vi "draw the stage.vi"(9 "angle":refnum<vi>, 10 "current pos...":refnum<vi>, 11 "XY Graph 2":refnum<vi>) -> ()   [LabVIEW 2018]
uses:
  cursor action.ctl
  generate linear region.vi
panel:
  out "angle 2":dbl(slide)=743.9484386624194 scale=-90.0..90.0 scale format="%^#6_6g"
  out "current pos...  2":dbl(slide) scale=0.0..16000.0
  in  "XY Graph":cluster{dbl[], dbl[]}[](graph)
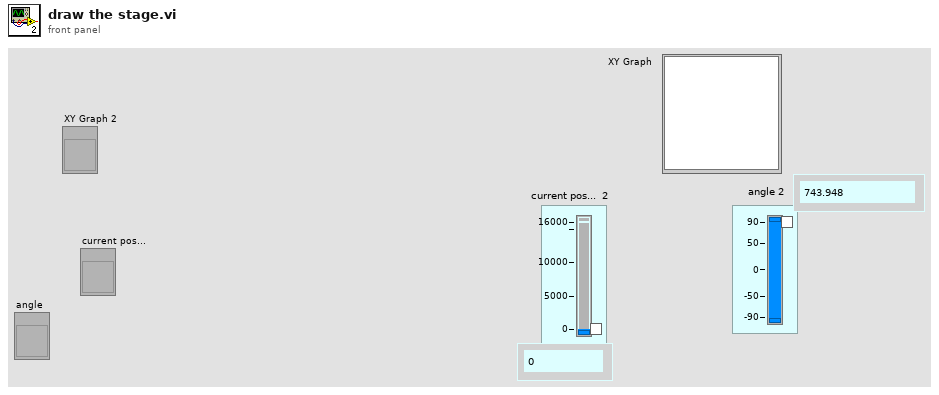
[diagram p1: front panel]
types:
  T1 = typedef "cursor action.ctl" = enum16{"range", "read", "write", "check", "zoom out", "smart zoom out", "zoom to aspect ratio 1", "zoom to win", "zoom out 20%", "zoom in 20%", "-empty", "smart zoom out&aspect", "move range left 20%", "move range right 20%", "move range up 20%", "move range down 20%", "zoom to X win", "zoom to Y win", "zoom out X", "zoom out Y", "zoom in X", "zoom in Y", "check plot scale"}
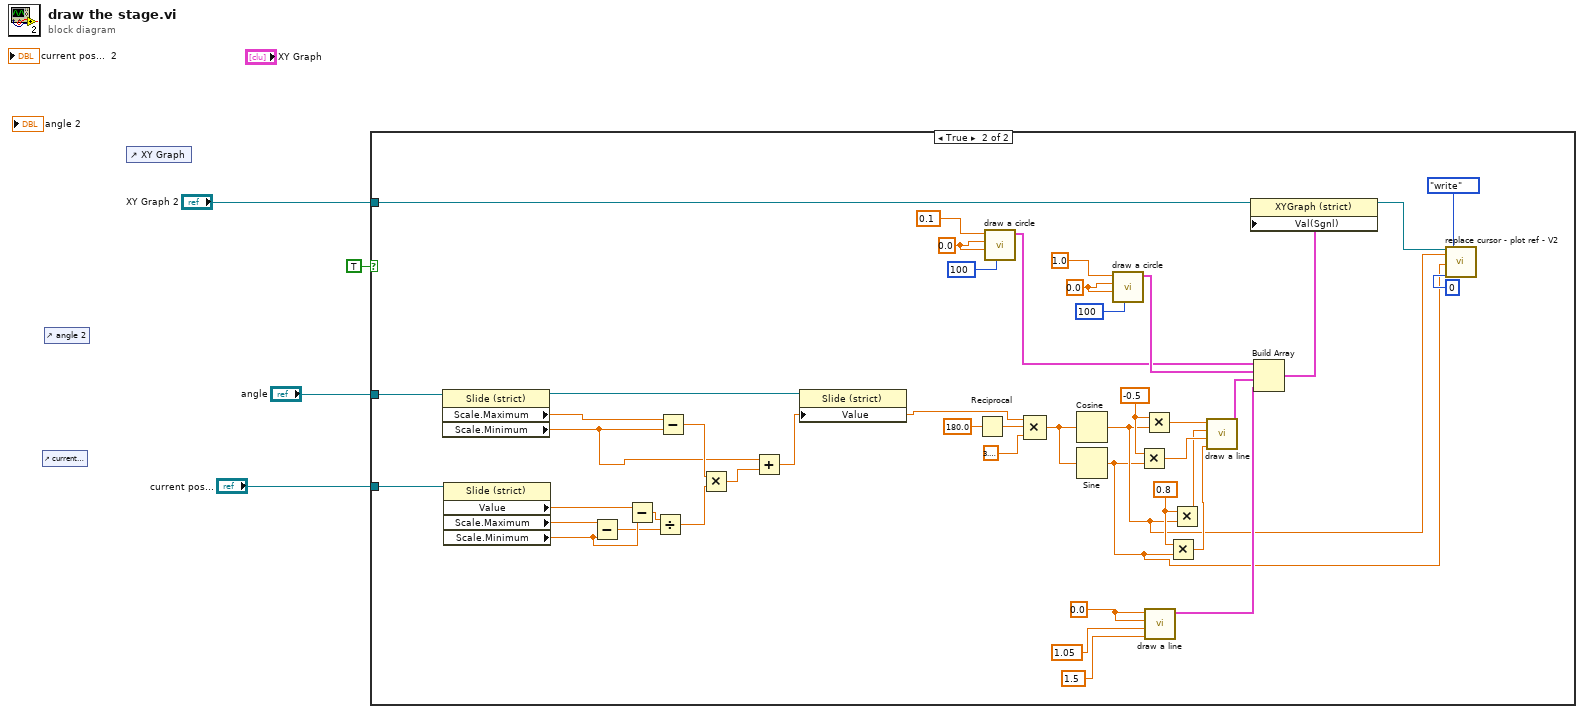
[diagram p0: block diagram]
diagram:
  n1 = control-ref of="current pos...  2"() -> ()  [unwired: 1 out]
  n2 = control-ref of="angle 2"() -> ()  [unwired: 1 out]
  n3 = control-ref of="XY Graph"() -> ()  [unwired: 1 out]
  n4 = case shown="True" TRUE {
    tunnel: "angle" -> [_ w47]
    tunnel: "current pos..." -> [_ w46]
    tunnel: "XY Graph 2" -> [_ w9]
    frame False {
    }
    frame True {
      w13 = 0.0 ("center x")
      w21 = 0.8 ("x")
      w23 = -0.5 ("x")
      w32 = 0.0 ("x0")
      w35 = 0.0 ("center x")
      n5 = property class="Slide (strict)"(reference=w47) -> (reference out=w36:refnum<vi>, "Scale.Maximum"=w40:dbl, "Scale.Minimum"=w14:dbl)  [unwired: 1 in, 1 out]
      n6 = property class="Slide (strict)"(reference=w46) -> ("Value"=w44:dbl, "Scale.Maximum"=w45:dbl, "Scale.Minimum"=w43:dbl)  [unwired: 1 in, 2 out]
      n7 = Subtract(x=w45, y=w43) -> (x-y=w41:dbl)
      n8 = Subtract(x=w44, y=w43) -> (x-y=w42:dbl)
      n9 = Divide(x=w42, y=w41) -> (x/y=w38:dbl)
      n10 = Subtract(x=w40, y=w14) -> (x-y=w39:dbl)
      n11 = Multiply(x=w39, y=w38) -> (x*y=w37:dbl)
      n12 = Add(x=w14, y=w37) -> (x+y=w26:dbl)
      n13 = property class="Slide (strict)"(reference=w36, "Value"=w26) -> ()  [unwired: 1 in, 2 out]
      n14 = Reciprocal(x=180.0 ("x0")) -> (1/x=w28:dbl)
      n15 = call "draw a circle.vi"("number of points"=100, "center Y"=w13, "center x"=w13, "radius"=0.1) -> ("output cluster"=w10:cluster{dbl[], dbl[]})  [unwired: 7 in]
      n16 = Compound Arithmetic op=MULTIPLY(w26, w28, 3.141592653589793) -> (w25:dbl)
      n17 = Cosine(x=w25) -> (cos(x)=w6:dbl)
      n18 = Sine(x=w25) -> (sin(x)=w5:dbl)
      n19 = call "draw a circle.vi"("number of points"=100, "center Y"=w35, "center x"=w35, "radius"=1.0) -> ("output cluster"=w18:cluster{dbl[], dbl[]})  [unwired: 7 in]
      n20 = Multiply(x=w23, y=w5) -> (x*y=w22:dbl)
      n21 = Multiply(x=w23, y=w6) -> (x*y=w24:dbl)
      n22 = call "draw a line.vi"("y1"=1.5 ("x0"), "y0"=1.05 ("x0"), "x1"=w32, "x0"=w32) -> ("output cluster"=w16:cluster{dbl[], dbl[]})  [unwired: 7 in]
      n23 = Multiply(x=w21, y=w5) -> (x*y=w19:dbl)
      n24 = Multiply(x=w21, y=w6) -> (x*y=w20:dbl)
      n25 = call "draw a line.vi"("y1"=w19, "y0"=w22, "x1"=w20, "x0"=w24) -> ("output cluster"=w17:cluster{dbl[], dbl[]})  [unwired: 7 in]
      n26 = Build Array(w10, w18, w17, w16) -> (w15:cluster{dbl[], dbl[]}[])
      n27 = property class="XYGraph (strict)"(reference=w9, "Val(Sgnl)"=w15) -> ()  [unwired: 1 in, 2 out]
      n28 = call "replace cursor - plot ref - V2.vi"("Plot ref in"=w9, "new X"=w6, "new  Y"=w5, "cursor index"=0, "cursor action"=cursor_action."write") -> ()  [unwired: 11 in, 4 out]
    }
  }
